vi "Get Type Specializations.vi"(8 "error in (no error)":errorcluster, 11 "MeasurementPluginService in":refnum<class "Measurement Plugin Service.lvclass">) -> (0 "error out":errorcluster, 2 "Type Specializations":T1[](array[typedef]), 3 "MeasurementPluginService out":refnum<class "Measurement Plugin Service.lvclass">)   [LabVIEW 2020, in "MeasurementLink Measurement Server.lvlib" / "Measurement Plugin Service.lvclass"]
uses:
  Measurement Plugin Service.lvclass
  Helpers/TypeDefs/Type Specialization.ctl
  MeasurementLink Measurement Server.lvlib
  Helpers/TypeDefs/Type Specialization Key.ctl
  Helpers/TypeDefs/Parameter Type Specialization.ctl
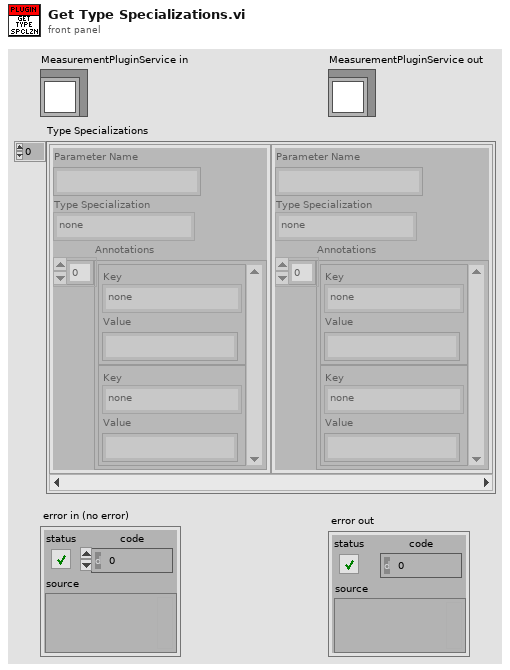
[diagram p1: front panel]
types:
  T1 = typedef "MeasurementLink Measurement Server.lvlib/Parameter Type Specialization.ctl" = cluster{"Parameter Name":string, "Type Specialization":T2, "Annotations":cluster{"Key":T3, "Value":string}[]}
  T2 = typedef "MeasurementLink Measurement Server.lvlib/Type Specialization.ctl" = enum16{"none", "pin", "path", "enum"}
  T3 = typedef "MeasurementLink Measurement Server.lvlib/Type Specialization Key.ctl" = enum16{"none", "pin.instrument_type", "enum.values"}
  T4 = typedef "MeasurementLink Measurement Server.lvlib/Measurement Plugin Service.lvclass/Plugin Paths.ctl" = cluster{"Get Measurement Details VI Path":path, "Get Type Specializations VI Path":path, "Get UI Details VI Path":path, "Measurement Logic VI Path":path, "Measurement Configuration CTL Path":path, "Measurement Results CTL Path":path}
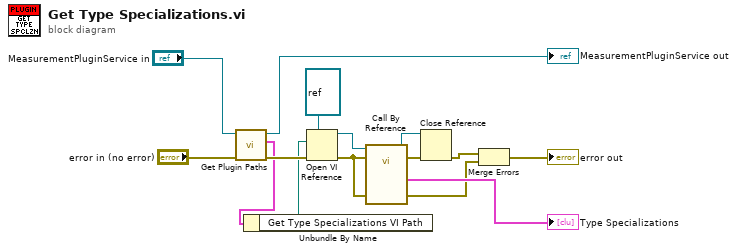
[diagram p0: block diagram]
diagram:
  n1 = call-dynamic "Get Plugin Paths.vi"("error in (no error)"="error in (no error)", "MeasurementPluginService in"="MeasurementPluginService in") -> ("error out"=w9:errorcluster, "Plugin Paths"=w1:T4, "MeasurementPluginService out"=→"MeasurementPluginService out":refnum<class "Measurement Plugin Service.lvclass">)  [unwired: 7 in]
  n2 = Unbundle By Name(w1) -> ("Get Type Specializations VI Path"=w8:path)
  n3 = Open VI Reference(type specifier VI Refnum (for type only)=refnum<vi> refnum, vi path=w8, error in (no error)=w9) -> (vi reference=w12:refnum<vi>, error out=w6:errorcluster)  [unwired: 3 in]
  n4 = call-by-ref "?"(reference=w12, error in=w6, 8:"error in (no error)"=w6) -> (reference out=w11:refnum<vi>, error out=w10:errorcluster, 0:"error out"=w2:errorcluster, "Type Specializations"=→"Type Specializations":T1[])  [unwired: 9 in]
  n5 = Close Reference(reference=w11, error in (no error)=w10) -> (error out=w4:errorcluster)
  n6 = Merge Errors(w4, w2) -> (→"error out":errorcluster)
